vi "niFpgaLrmPalette_MergeVI_Register.vi"   [LabVIEW 2017]
doc: "Represents a VI-defined register item. Right-click the node and select <B>Configure</B> to configure the VI-defined register item."
uses:
  <vilib>/rvi/DataTransferAndStorage/Container/Common/niFpgaContainerGetUniqueNameForEmu.vi
  <vilib>/rvi/DataTransferAndStorage/Container/Common/niFpgaContainerSetEmuInfo.vi
  <vilib>/rvi/eio/common/nirviEmuReportErrorAndStop.vi
  <vilib>/rvi/LocalResourceManager/LocalResourceManager.xnode
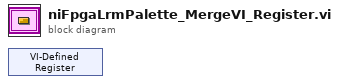
[diagram p0: block diagram]
diagram:
  n1 = xnode "VI-Defined Register"() -> ()  [unwired: 1 out]
